vi "GetNumericType.vi"(6 "error in":errorcluster, 9 "Numeric in":refnum<class "Numeric.lvclass">) -> (0 "error out":errorcluster, 3 "Numeric out":refnum<class "Numeric.lvclass">, 4 "String":string)   [LabVIEW 2014, in "Numeric.lvclass"]
uses:
  Numeric.lvclass
  Control/Control.lvclass/Control.ctl
  Control/Control.lvclass
  <vilib>/Utility/VariantDataType/VariantType.lvlib
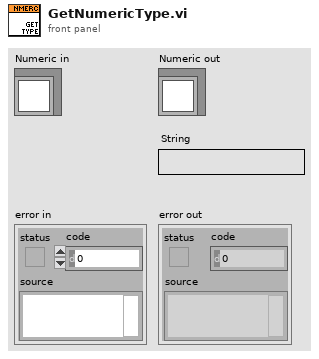
[diagram p1: front panel]
types:
  T1 = typedef "LVNumericRepresentation.ctl" = enum32{"Extended Precision", "Double Precision", "Single Precision", "Long", "Word", "Byte", "Unsigned Long", "Unsigned Word", "Unsigned Byte", "Complex Extended", "Complex Double", "Complex Single", "Quad", "Unsigned Quad", "Fixed-Point"}
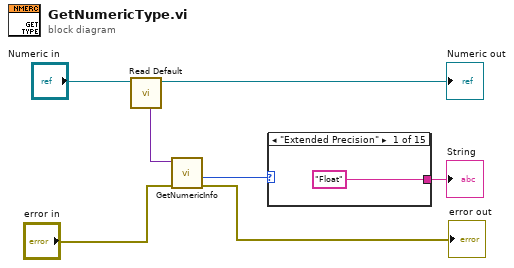
[diagram p0: block diagram]
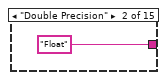
[diagram p2: hidden frame]
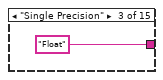
[diagram p3: hidden frame]
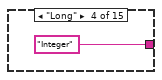
[diagram p4: hidden frame]
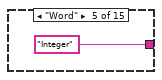
[diagram p5: hidden frame]
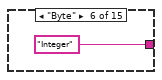
[diagram p6: hidden frame]
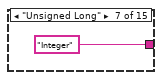
[diagram p7: hidden frame]
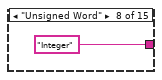
[diagram p8: hidden frame]
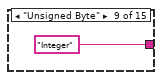
[diagram p9: hidden frame]
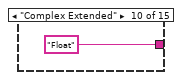
[diagram p10: hidden frame]
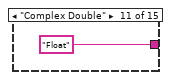
[diagram p11: hidden frame]
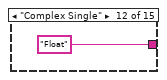
[diagram p12: hidden frame]
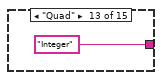
[diagram p13: hidden frame]
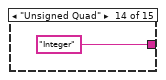
[diagram p14: hidden frame]
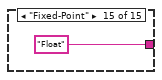
[diagram p15: hidden frame]
diagram:
  n1 = call "Read Default.vi"("Control in"="Numeric in") -> ("Control out"=→"Numeric out":refnum<class "Numeric.lvclass">, "Default"=w6:variant)  [unwired: 7 in]
  n2 = call <vilib>:"GetNumericInfo.vi"("error in (no error)"="error in", "Variant"=w6) -> ("error out"=→"error out":errorcluster, "representation"=w5:T1)  [unwired: 6 in, 2 out]
  n3 = case shown="\"Extended Precision\"" w5 {
    tunnel: ["Float" "Float" "Float" "Integer" "Integer" "Integer" "Integer" "Integer" "Integer" "Float" "Float" "Float" "Integer" "Integer" "Float"] -> w4
    frame "Extended Precision" {
    }
    frame "Double Precision" {
    }
    frame "Single Precision" {
    }
    frame "Long" {
    }
    frame "Word" {
    }
    frame "Byte" {
    }
    frame "Unsigned Long" {
    }
    frame "Unsigned Word" {
    }
    frame "Unsigned Byte" {
    }
    frame "Complex Extended" {
    }
    frame "Complex Double" {
    }
    frame "Complex Single" {
    }
    frame "Quad" {
    }
    frame "Unsigned Quad" {
    }
    frame "Fixed-Point" {
    }
  }
  "String" <- w4
